vi "Close Web Service.vi"(8 "error in (no error)":errorcluster caption="错误输入（无错误）", 11 "EEPromCodeService 引用句柄":refnum<k24>) -> (0 "error out":errorcluster caption="错误输出")   [LabVIEW 2011]
uses:
  Data/EEPromCodeService.dll
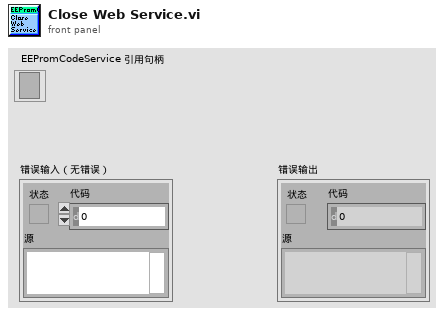
[diagram p1: front panel]
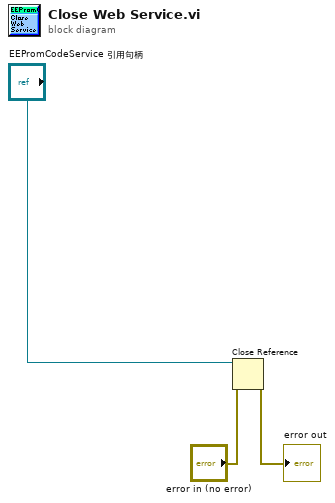
[diagram p0: block diagram]
diagram:
  n1 = Close Reference(reference="EEPromCodeService 引用句柄", error in (no error)="error in (no error)") -> (error out=→"error out":errorcluster)
